vi "Read Worker Type.vi"(8 "error in (no error)":errorcluster, 11 "Barista in":refnum<class "Barista.lvclass">) -> (0 "error out":errorcluster, 2 "Type":string, 3 "Barista out":refnum<class "Barista.lvclass">)   [LabVIEW 2023, in "Barista.lvclass"]
doc: "Returns the type of worker. This method is required by any descendant of the Worker class.\n\nBecause this method is implemented by the Barista class, it will always return \"Barista.\""
uses:
  Barista.lvclass
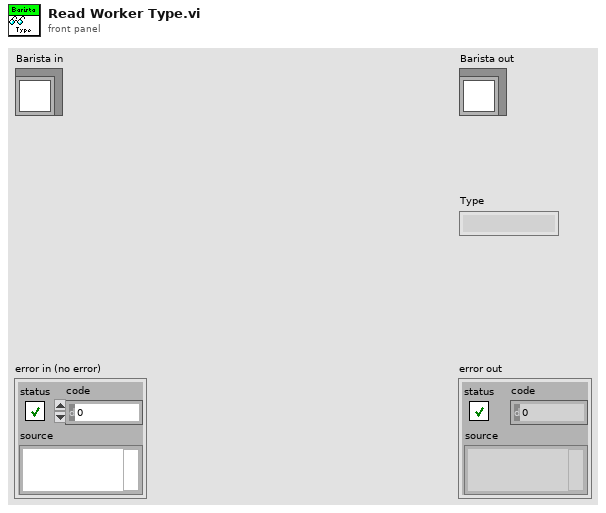
[diagram p1: front panel]
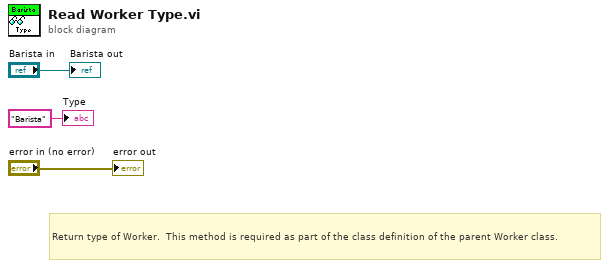
[diagram p0: block diagram]
diagram:
  # "Return type of Worker.  This method is required as part of the class definition of the parent Worker class."
  "error out" <- "error in (no error)"
  "Barista out" <- "Barista in"
  "Type" <- "Barista" ("Type")
